vi "MDrive_Send_Command.vi"(4 "error in":errorcluster, 5 "Send String":string, 7 "VISA resource name in":refnum<visa-resource-name>) -> (0 "error out":errorcluster, 1 "read buffer":string, 3 "VISA resource name out":refnum<visa-resource-name>)   [LabVIEW 2017]
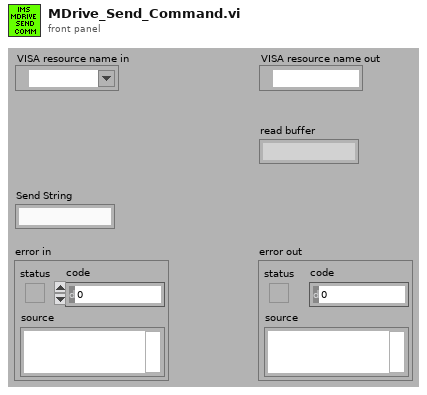
[diagram p1: front panel]
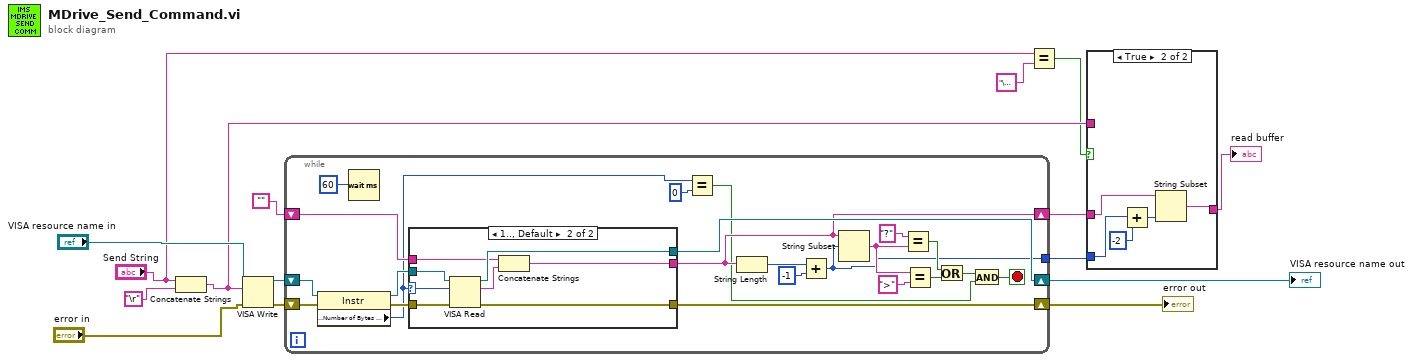
[diagram p0: block diagram]
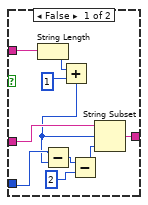
[diagram p2: hidden frame]
diagram:
  n1 = Concatenate Strings("Send String", "\r") -> (w5:string)
  n2 = VISA Write(VISA resource name="VISA resource name in", write buffer=w5, error in (no error)="error in") -> (VISA resource name out=w14:refnum<visa-resource-name>, error out=w13:errorcluster)  [unwired: 1 out]
  n3 = while {
    shift-right: [w28] -> w12
    shift-left: "" -> [w33]
    shift-right: [w34] -> w8
    shift-left: w14 -> [w32]
    shift-right: [w35] -> w9
    shift-left: w13 -> [w31]
    tunnel: [w17] -> w4
    stop <- w18 stop-if-true
    n4 = property class="Instr"(reference=w32, error in=w31) -> (reference out=w36:refnum<visa-resource-name>, error out=w37:errorcluster, "Serial Settings:Number of Bytes at Serial Port"=w30:u32)
    n5 = Wait (ms)(milliseconds to wait=u32 60) -> ()  [unwired: 1 out]
    n6 = case shown="1.., Default" w30 {
      selector: w30 -> [_ w46]
      tunnel: w37 -> [w39 w48]
      tunnel: w36 -> [w40 w47]
      tunnel: [w39 w45] -> w35
      tunnel: [w40 w44] -> w34
      tunnel: w33 -> [w38 w43]
      tunnel: [w38 w42] -> w28
      frame 0 {
      }
      frame 1.., Default {
        n7 = VISA Read(VISA resource name=w47, byte count=w46, error in (no error)=w48) -> (VISA resource name out=w44:refnum<visa-resource-name>, read buffer=w41:string, error out=w45:errorcluster)  [unwired: 1 out]
        n8 = Concatenate Strings(w43, w41) -> (w42:string)
      }
    }
    n9 = Equal?(x=w30, y=u32 0) -> (x = y?=w24:bool)
    n10 = String Length(string=w28) -> (length=w26:i32)
    n11 = Add(x=w26, y=-1 ("offset (0)")) -> (x+y=w17:i32)
    n12 = String Subset(string=w28, offset (0)=w17) -> (substring=w23:string)  [unwired: 1 in]
    n13 = Equal?(x="?", y=w23) -> (x = y?=w22:bool)
    n14 = Equal?(x=w23, y=">") -> (x = y?=w21:bool)
    n15 = Or(x=w22, y=w21) -> (x .or. y?=w19:bool)
    n16 = And(x=w19, y=w24) -> (x .and. y?=w18:bool)
  }
  "error out" <- w9
  "VISA resource name out" <- w8
  n17 = Equal?(x="Send String", y="\u0003") -> (x = y?=w1:bool)
  n18 = case shown="True" w1 {
    tunnel: w12 -> [w58 w62]
    tunnel: [w57 w63] -> w6
    tunnel: w5 -> [w56 _]
    tunnel: w4 -> [w55 w60]
    frame False {
      n19 = String Length(string=w56) -> (length=w54:i32)
      n20 = Add(x=w54, y=1) -> (x+y=w53:i32)
      n21 = Subtract(x=w55, y=w53) -> (x-y=w51:i32)
      n22 = Subtract(x=w51, y=2) -> (x-y=w50:i32)
      n23 = String Subset(string=w58, offset (0)=w53, length (rest)=w50) -> (substring=w57:string)
    }
    frame True {
      n24 = Add(x=w60, y=-2 ("offset (0)")) -> (x+y=w59:i32)
      n25 = String Subset(string=w62, length (rest)=w59) -> (substring=w63:string)  [unwired: 1 in]
    }
  }
  "read buffer" <- w6
